vi "S2DS_External Control (SubVI).vi"(8 "error in (no error)":errorcluster, 10 "Timeout (ms), Check interval (ms)":i32[](array[numeric])) -> (0 "error out":errorcluster)   [LabVIEW 2025]
uses:
  <vilib>/Utility/config.llb/Write Key (String).vi
  <vilib>/Utility/config.llb/Read Key (String).vi
  <vilib>/Utility/config.llb/NI_LVConfig.lvlib
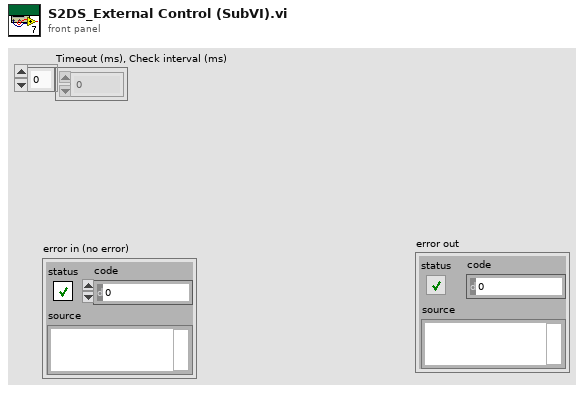
[diagram p1: front panel]
types:
  T1 = typedef "NI_LVConfig.lvlib/Config Data RefNum.ctl" = refnum<k1>
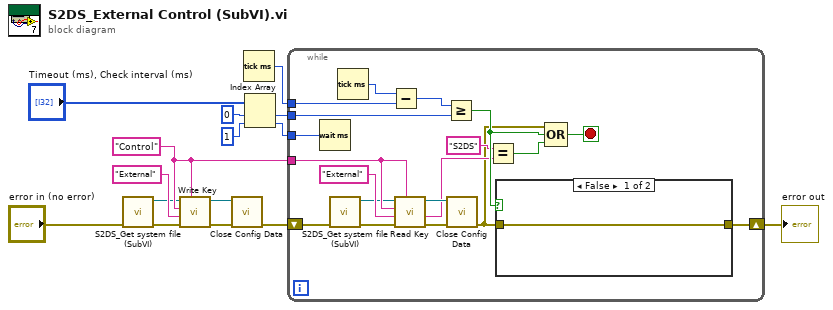
[diagram p0: block diagram]
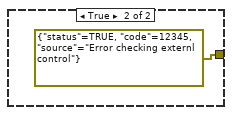
[diagram p2: hidden frame]
diagram:
  w9 = "Control"
  n1 = call "S2DS_Get system file (SubVI).vi"("error in (no error)"="error in (no error)") -> ("error out"=w2:errorcluster, "Refnum out"=w3:T1)  [unwired: 9 in]
  n2 = call-poly <vilib>:"Write Key.vi"("section"=w9, "error in (no error)"=w2, "value"="External", "key"=w9, "refnum"=w3) -> ("error out"=w12:errorcluster, "refnum out"=w13:T1)  [unwired: 4 in, 1 out]
  n3 = call <vilib>:"Close Config Data.vi"("error in (no error)"=w12, "refnum"=w13) -> ("error out"=w11:errorcluster)  [unwired: 8 in, 1 out]
  n4 = Tick Count (ms)() -> (millisecond timer value=w15:u32)
  n5 = Index Array(array="Timeout (ms), Check interval (ms)", index #1=0 ("index"), index #2=1 ("index")) -> (element #1=w5:i32, element #2=w4:i32)
  n6 = while {
    tunnel: w9 -> [w25]
    shift-right: [w26] -> w14
    shift-left: w11 -> [w18]
    tunnel: w15 -> [w33]
    tunnel: w5 -> [w31]
    tunnel: w4 -> [w19]
    stop <- w30 stop-if-true
    n7 = Wait (ms)(milliseconds to wait=w19) -> ()  [unwired: 1 out]
    n8 = call "S2DS_Get system file (SubVI).vi"("error in (no error)"=w18) -> ("error out"=w17:errorcluster, "Refnum out"=w16:T1)  [unwired: 9 in]
    n9 = Tick Count (ms)() -> (millisecond timer value=w34:u32)
    n10 = Subtract(x=w34, y=w33) -> (x-y=w32:u32)
    n11 = call-poly <vilib>:"Read Key.vi"("section"=w25, "error in (no error)"=w17, "default value"="External", "key"=w25, "refnum"=w16) -> ("error out"=w28:errorcluster, "value"=w24:string, "refnum out"=w29:T1)  [unwired: 3 in, 1 out]
    n12 = Greater Or Equal?(x=w32, y=w31) -> (x >= y?=w27:bool)
    n13 = call <vilib>:"Close Config Data.vi"("error in (no error)"=w28, "refnum"=w29) -> ("error out"=w20:errorcluster)  [unwired: 8 in, 1 out]
    n14 = Equal?(x="S2DS", y=w24) -> (x = y?=w22:bool)
    n15 = case shown="False" w27 {
      tunnel: w20 -> [w35 _]
      tunnel: [w35 errorcluster {"status"=TRUE, "code"=12345, "source"="Error checking externl control"} ("error out")] -> w26
      frame False {
      }
      frame True {
      }
    }
    n16 = Compound Arithmetic op=OR(w20, w27, w22) -> (w30:bool)
  }
  "error out" <- w14
